vi "Determine which Throws Need Parallel Calc.vi"() -> ()   [LabVIEW 2013]
uses:
  Controls/USID.ctl
panel:
  out "Array 2":dbl[](array[numeric])
  out "Array":dbl[](array[numeric])
  in  "USID":T1 max=15
  in  "Individial_R_Measurements":dbl[](array[numeric])
  in  "Pins_To_Test":string[](array[string])=["RF1", "RF4", "RF2", "RF3"]
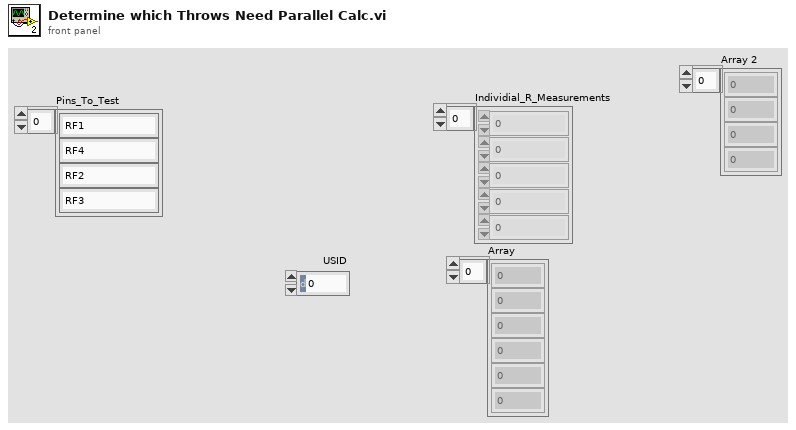
[diagram p1: front panel]
types:
  T1 = typedef "USID.ctl" = u8
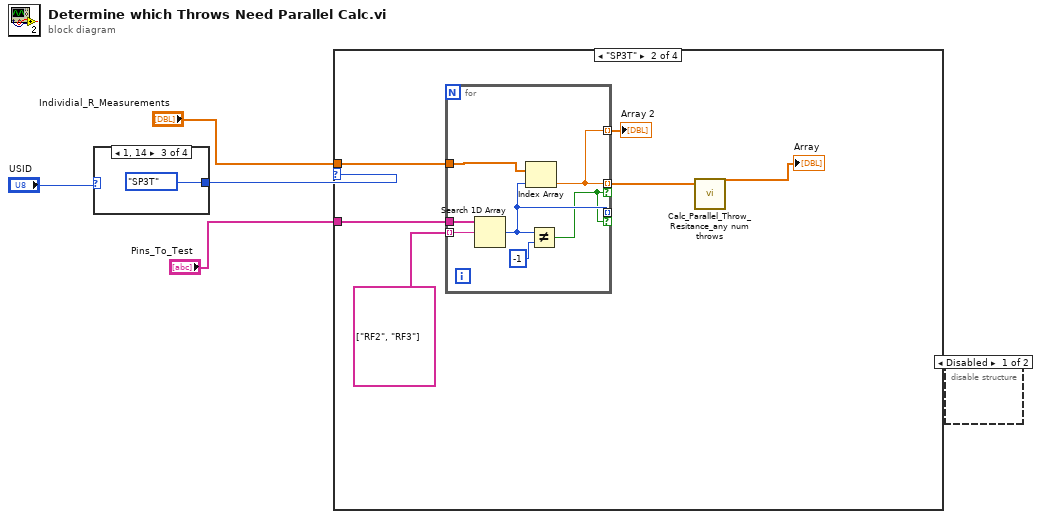
[diagram p0: block diagram]
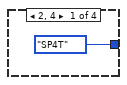
[diagram p3: hidden frame]
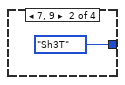
[diagram p4: hidden frame]
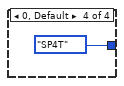
[diagram p5: hidden frame]
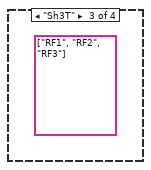
[diagram p7: hidden frame]
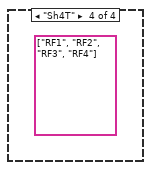
[diagram p8: hidden frame]
diagram:
  n1 = case shown="1, 14" "USID" {
    tunnel: [enum16{"SP4T", "SP3T", "Sh3T", "Sh4T"}."SP4T" ("Die Type 2") enum16{"SP4T", "SP3T", "Sh3T", "Sh4T"}."Sh3T" ("Die Type 2") enum16{"SP4T", "SP3T", "Sh3T", "Sh4T"}."SP3T" ("Die Type 2") enum16{"SP4T", "SP3T", "Sh3T", "Sh4T"}."SP4T" ("Die Type 2")] -> w3
    frame 2, 4 {
    }
    frame 7, 9 {
    }
    frame 1, 14 {
    }
    frame 0, Default {
    }
  }
  n2 = case shown="\"SP3T\"" w3 {
    tunnel: "Pins_To_Test" -> [_ w14 _ _]
    tunnel: "Individial_R_Measurements" -> [_ w10 _ _]
    frame "SP4T", Default {
    }
    frame "SP3T" {
      n3 = for {
        tunnel: [w15] -> w12 mode=indexing if=w16
        tunnel: w14 -> [w21]
        tunnel: w10 -> [w18]
        tunnel: string[] ["RF2", "RF3"] ("Pins_To_Publish") -> [w20] mode=indexing
        tunnel: [w17] -> _ mode=indexing if=w16
        tunnel: [w15] -> w9 mode=indexing
        n4 = Search 1D Array(1D array=w21, element=w20) -> (index of element=w17:i32)  [unwired: 1 in]
        n5 = Index Array(array=w18, index=w17) -> (element=w15:dbl)
        n6 = Not Equal?(x=w17, y=-1) -> (x != y?=w16:bool)
      }
      "Array 2" <- w9
      n7 = call "Calc_Parallel_Throw_Resitance_any num throws.vi"("Resitance_Per Site"=w12) -> ("Parallel_Resitance"=→"Array":dbl[])  [unwired: 10 in]
    }
    frame "Sh3T" {
      (unwired) string[] ["RF1", "RF2", "RF3"] ("Pins_To_Publish")
    }
    frame "Sh4T" {
      (unwired) string[] ["RF1", "RF2", "RF3", "RF4"] ("Pins_To_Publish")
    }
  }
  n8 = disable-structure shown="Disabled" {
    frame Disabled {
    }
    frame Enabled {
    }
  }
